vi "Get Reference.vi"(8 "Error In":errorcluster, 11 "Logger In":refnum<class "LoggerAPI.lvclass">) -> (0 "Error Out":errorcluster, 2 "Reference":refnum<class "ILogger.lvclass">, 3 "Logger Out":refnum<class "LoggerAPI.lvclass">)   [LabVIEW 2020, in "LoggerAPI.lvclass"]
uses:
  LoggerAPI.lvclass
  ILogger/ILogger.lvclass
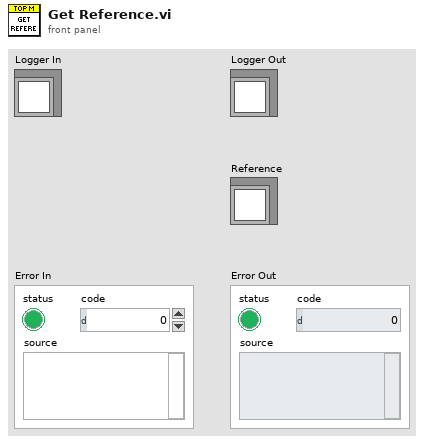
[diagram p1: front panel]
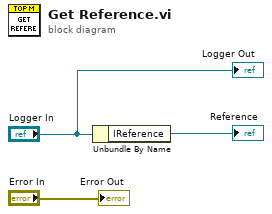
[diagram p0: block diagram]
diagram:
  n1 = Unbundle By Name("Logger In") -> ("IReference"=→"Reference":refnum<class "ILogger.lvclass">)
  "Logger Out" <- "Logger In"
  "Error Out" <- "Error In"
